vi "SQLite Delete All or One SensorConfig Data.vi"(6 "sadfads":enum16{"DeleteAll", "DeleteOne"}(ring), 7 "Main":string="0", 8 "error in (no error)":errorcluster, 11 "VariableName":string) -> (0 "error out":errorcluster, 3 "VariableName Out":string, 5 "Main Out":string)   [LabVIEW 2017, in "SQLite.lvclass"]
doc: "根据Main 和Variable的名称，在保存新的校准值之前删除所有的旧数据。\n2015-11-03 15:56:09\n蒋松\njiangsong@outlook.com"
uses:
  SQLite.lvclass
  SQLiteFileName.ctl
  TabelFullName.ctl
  <userlib>/LabSQL/LabSQL.lvlib
panel:
  in  "error in (no error) 2":errorcluster
  out "Select SQL CMD":string
  # "sfdgs\nsfdgs"
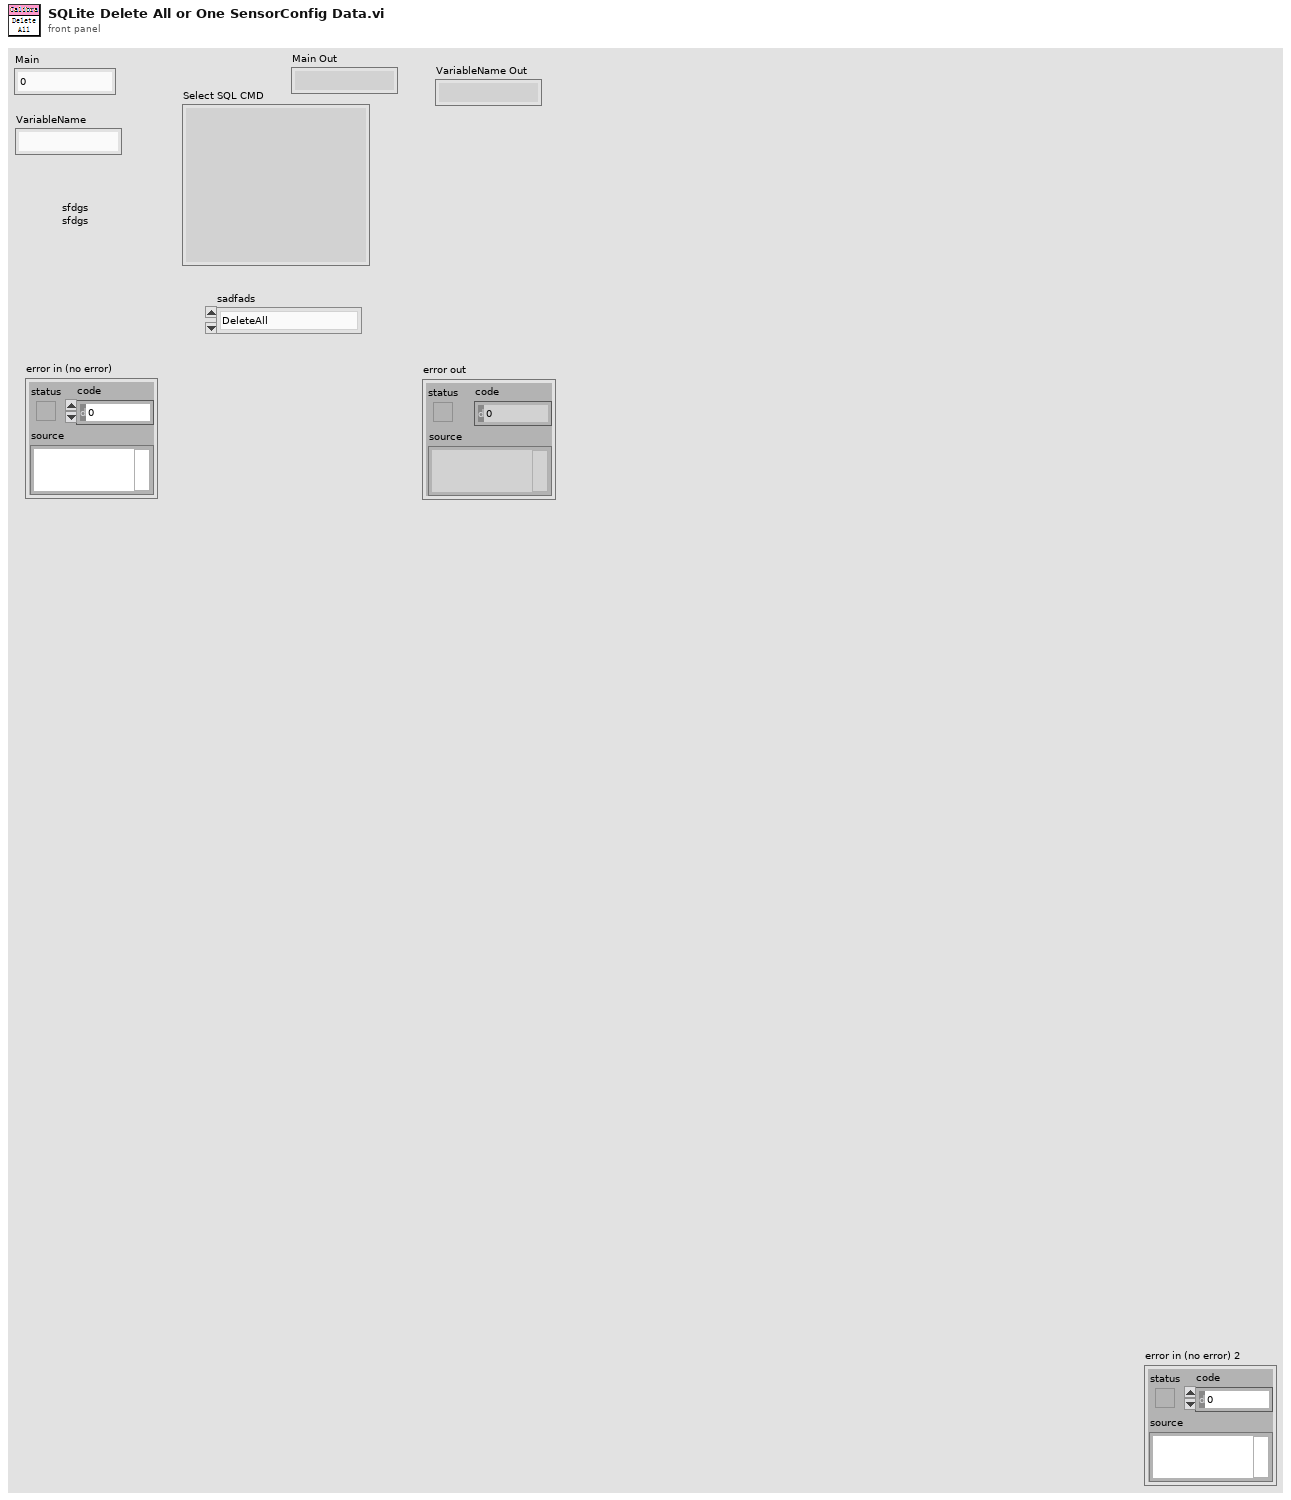
[diagram p1: front panel]
types:
  T1 = typedef "SQLite.lvclass/TabelFullName.ctl" = string
  T2 = typedef "SQLite.lvclass/SQLiteFileName.ctl" = string
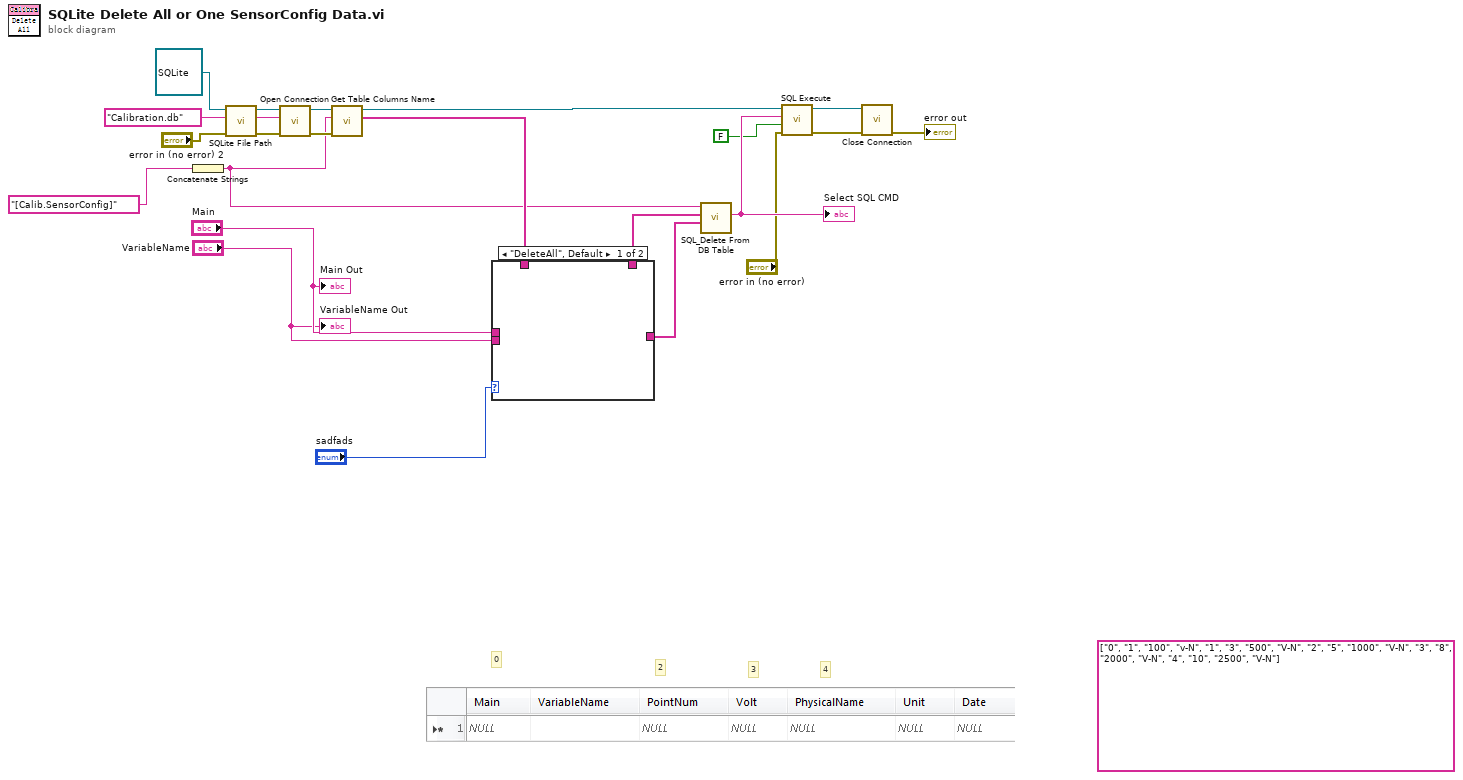
[diagram p0: block diagram]
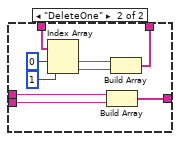
[diagram p2: hidden frame]
diagram:
  (unwired) string[][] [["0", "1", "100", "v-N"], ["1", "3", "500", "V-N"], ["2", "5", "1000", "V-N"], ["3", "8", "2000", "V-N"], ["4", "10", "2500", "V-N"]] ("Result Set 2")
  # "3"
  # "0"
  # "2"
  # "4"
  n1 = Concatenate Strings(T1 "[Calib.SensorConfig]" ("TabelFullName")) -> (w10:string)
  n2 = call "SQLite File Path.vi"("error in (no error)"="error in (no error) 2", "SQLiteFileName"=T2 "Calibration.db", "SQLite in"=refnum<class "SQLite.lvclass"> refnum ("SQLite.lvclass")) -> ("error out"=w12:errorcluster, "string"=w16:string, "SQLite out"=w14:refnum<class "SQLite.lvclass">)  [unwired: 6 in]
  n3 = call-dynamic "Open Connection.vi"("error in (no error)"=w12, "ConnectionString"=w16, "HostDB in"=w14) -> ("error out"=w17:errorcluster, "HostDB out"=w18:refnum<class "SQLite.lvclass">)  [unwired: 7 in]
  n4 = call-dynamic "Get Table Columns Name.vi"("error in (no error)"=w17, "TableName"=w10, "HostDB in"=w18) -> ("ColunmsList"=w11:string[], "HostDB out"=w9:refnum<class "SQLite.lvclass">)  [unwired: 4 in, 3 out]
  n5 = case shown="\"DeleteAll\", Default" "sadfads" {
    tunnel: "Main" -> [_ w32]
    tunnel: "VariableName" -> [_ w31]
    tunnel: [_ w30] -> w21
    tunnel: [_ w25] -> w20
    tunnel: w11 -> [_ w24]
    frame "DeleteAll", Default {
    }
    frame "DeleteOne" {
      n6 = Index Array(array=w24, index #1=0 ("index"), index #2=1 ("index")) -> (element #1=w28:string, element #2=w29:string)
      n7 = Build Array(w32, w31) -> (w25:string[])
      n8 = Build Array(w28, w29) -> (w30:string[])
    }
  }
  n9 = call <userlib>:"SQL_Delete From DB Table.vi"("ColumnsValue"=w20, "ColumnsNameList"=w21, "TableName"=w10) -> ("Select SQL CMD"=w6:string)  [unwired: 8 in]
  "Select SQL CMD" <- w6
  n10 = call-dynamic "SQL Execute.vi"("error in (no error)"="error in (no error)", "Return Data (T)"=FALSE, "Command Text"=w6, "HostDB in"=w9) -> ("error out"=w7:errorcluster, "HostDB out"=w8:refnum<class "SQLite.lvclass">)  [unwired: 3 in, 3 out]
  n11 = call-dynamic "Close Connection.vi"("error in (no error)"=w7, "HostDB in"=w8) -> ("error out"=→"error out":errorcluster)  [unwired: 8 in, 1 out]
  "VariableName Out" <- "VariableName"
  "Main Out" <- "Main"
